vi "Solution part 2.vi"(11 "data?":bool) -> ()   [LabVIEW 2020]
panel:
  in  "manual input":string
  in  "file input?":bool
  out "Timestamp":u64
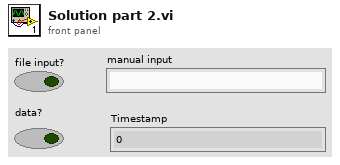
[diagram p1: front panel]
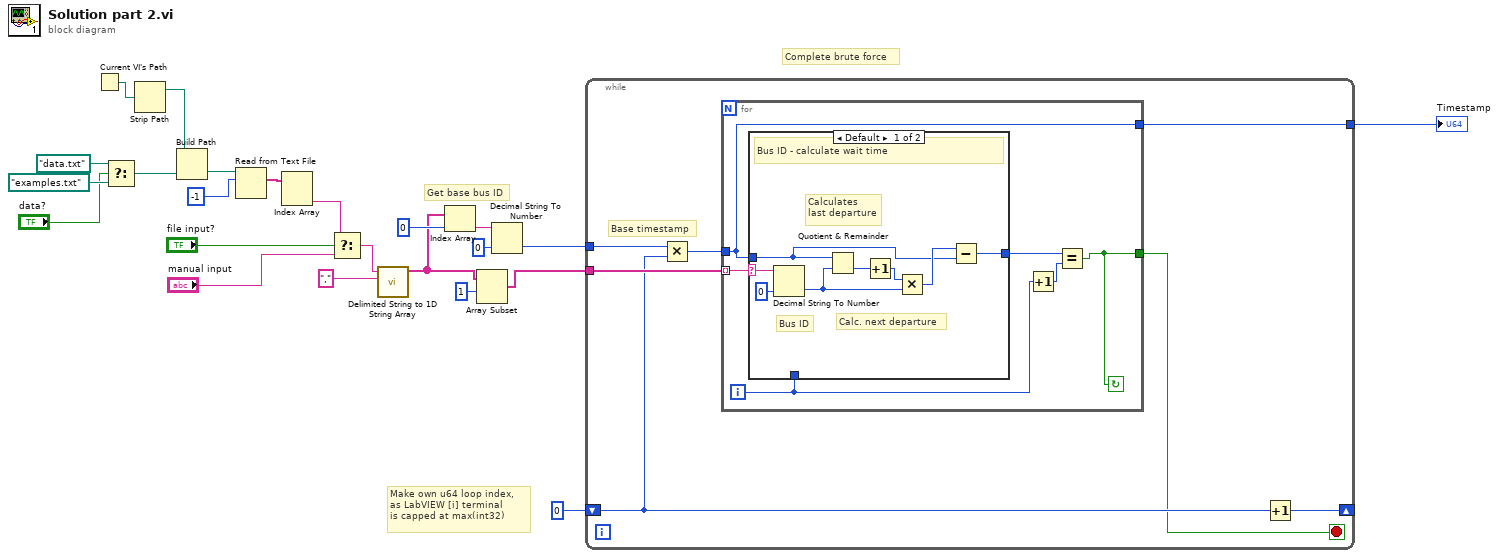
[diagram p0: block diagram]
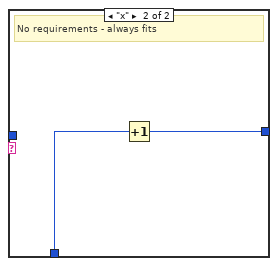
[diagram p2: hidden frame]
diagram:
  # "Complete brute force"
  # "Make own u64 loop index,\nas LabVIEW [i] terminal\nis capped at max(int32)"
  # "Get base bus ID"
  n1 = Current VI's Path() -> (path=w20:path)
  n2 = Select(t=path "data.txt", s="data?", f=path "examples.txt") -> (s? t:f=w21:path)
  n3 = Strip Path(path=w20) -> (stripped path=w19:path)  [unwired: 1 out]
  n4 = Build Path(base path=w19, name or relative path=w21) -> (appended path=w18:path)
  n5 = Read from Text File(file (use dialog)=w18, count=-1) -> (text=w15:string[])  [unwired: 2 in, 3 out]
  n6 = Index Array(array=w15) -> (element #2=w14:string)  [unwired: 2 in, 1 out]
  n7 = Select(t=w14, s="file input?", f="manual input") -> (s? t:f=w3:string)
  n8 = call <vilib>:"Delimited String to 1D String Array.vi"("delimiter"=",", "delimited string"=w3) -> ("string array"=w6:string[])  [unwired: 9 in]
  n9 = Index Array(array=w6, index=0) -> (element=w11:string)
  n10 = Array Subset(array=w6, index=1) -> (w7:string[])  [unwired: 1 in]
  n11 = Decimal String To Number(string=w11, default (0L)=u64 0 ("index")) -> (number=w10:u64)  [unwired: 1 in, 1 out]
  n12 = while {
    tunnel: w7 -> [w30]
    tunnel: w10 -> [w28]
    shift-right: [w29] -> _
    shift-left: u64 0 ("index") -> [w27]
    tunnel: [w24] -> w4
    stop <- w25 stop-if-true
    # "Base timestamp"
    n13 = Multiply(x=w28, y=w27) -> (x*y=w26:u64)
    n14 = for {
      tunnel: w30 -> [w36] mode=indexing
      tunnel: [w34] -> w25
      tunnel: w26 -> [w31]
      tunnel: [w31] -> w24
      i -> [w32]
      stop <- w34 continue-if-true
      n15 = case shown="Default" w36 {
        selector: w36 -> [w44 _]
        tunnel: [w39 w45] -> w35
        tunnel: w31 -> [w37 _]
        tunnel: w32 -> [_ w46]
        frame Default {
          # "Bus ID"
          # "Calc. next departure"
          # "Calculates \nlast departure"
          # "Bus ID - calculate wait time"
          n16 = Decimal String To Number(string=w44, default (0L)=u64 0 ("index")) -> (number=w42:u64)  [unwired: 1 in, 1 out]
          n17 = Quotient & Remainder(x=w37, y=w42) -> (floor(x/y)=w43:u64)  [unwired: 1 out]
          n18 = Increment(x=w43) -> (x+1=w41:u64)
          n19 = Multiply(x=w41, y=w42) -> (x*y=w40:u64)
          n20 = Subtract(x=w40, y=w37) -> (x-y=w39:u64)
        }
        frame "x" {
          # "No requirements - always fits"
          n21 = Increment(x=w46) -> (x+1=w45:i32)
        }
      }
      n22 = Increment(x=w32) -> (x+1=w33:i32)
      n23 = Equal?(x=w35, y=w33) -> (x = y?=w34:bool)
    }
    n24 = Increment(x=w27) -> (x+1=w29:u64)
  }
  "Timestamp" <- w4
